vi "Remote1POV.vi"() -> (0 "POV":T1 items=["None"=-1, "POV Up"=0, "POV Up Right"=1, "POV Right"=2, "POV Down Right"=3, "POV Down"=4, "POV Down Left"=5, "POV Left"=6, "POV Up Left"=7])   [LabVIEW 2010, in "FTC.lvlib" / "Remote Interface.lvlib"]
uses:
  Remote Interface.lvlib
  <vilib>/FTC/FTC POVState.ctl
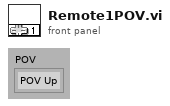
[diagram p1: front panel]
types:
  T1 = typedef "FTC POVState.ctl" = i8
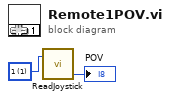
[diagram p0: block diagram]
diagram:
  w1 = u8 1 items=["1"=1, "2"=2] ("Joystick Number (1)")
  n1 = call "ReadJoystick.vi"("Remote (1)"=w1) -> ("POV"=→"POV":T1)  [unwired: 1 in, 2 out]
